vi "create default alias.vi"(8 "error in":errorcluster, 11 "configuration in":refnum<class "Standard Engine Configuration.lvclass">) -> (0 "error out":errorcluster, 2 "default alias":string, 3 "configuration out":refnum<class "Standard Engine Configuration.lvclass">)   [LabVIEW 2013, in "Standard Engine Configuration.lvclass"]
uses:
  Standard Engine Configuration.lvclass
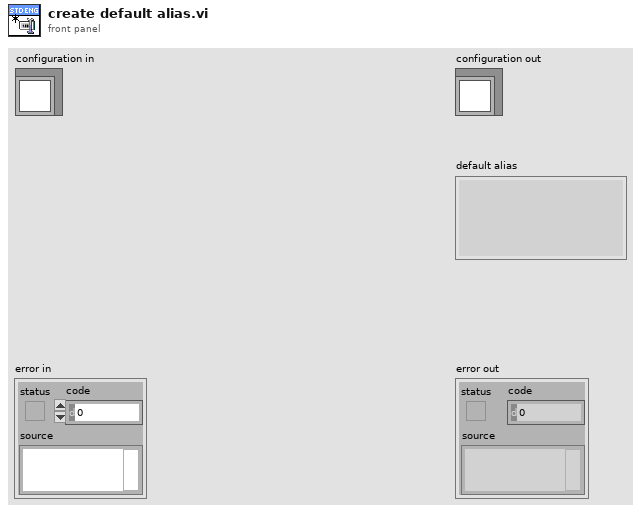
[diagram p1: front panel]
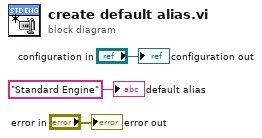
[diagram p0: block diagram]
diagram:
  "error out" <- "error in"
  "configuration out" <- "configuration in"
  "default alias" <- "Standard Engine" ("default alias")
